vi "Write.vi"(8 "error in (no error)":errorcluster, 10 "Input":variant, 11 "DAQmx DIO in":refnum<class "DAQmx DIO.lvclass">) -> (0 "error out":errorcluster, 3 "DAQmx DIO out":refnum<class "DAQmx DIO.lvclass">)   [LabVIEW 2017, in "DAQmx DIO.lvclass"]
uses:
  DAQmx DIO.lvclass
  C:/Microcellular Plastics Lab/Hardware Settings/Hardware Types/DAQmx/DAQmx.lvclass
  DAQmx/DAQmx.lvclass/DAQmx.ctl
  <vilib>/DAQmx/write.llb/DAQmx Write (Digital 1D Bool NChan 1Samp 1Line).vi
  DAQmx/Accessors/Read DAQmx Task Name.vi
  <vilib>/DAQmx/miscellaneous.llb/DAQmx Fill In Error Info.vi
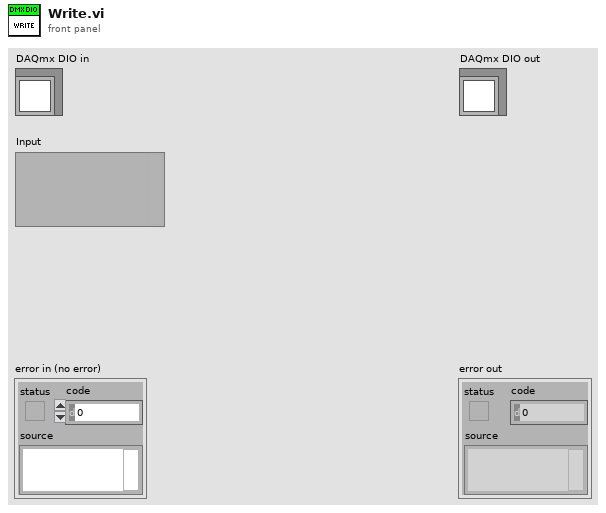
[diagram p1: front panel]
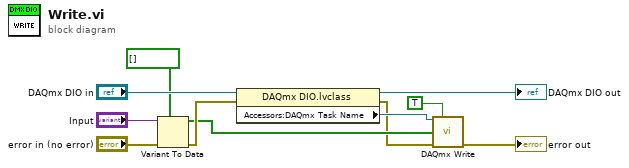
[diagram p0: block diagram]
diagram:
  n1 = Variant To Data(error in="error in (no error)", type=bool[] [], Variant="Input") -> (data=w3:bool[], error out=w7:errorcluster)
  n2 = property class="DAQmx DIO.lvclass"(reference="DAQmx DIO in", error in=w7) -> (reference out=→"DAQmx DIO out":refnum<class "DAQmx DIO.lvclass">, error out=w2:errorcluster, "Accessors:DAQmx Task Name"=w6:refnum<k21>)
  n3 = call-poly <vilib>:"DAQmx Write.vi"("task/channels in"=w6, "auto start"=TRUE, "data"=w3, "error in"=w2) -> ("error out"=→"error out":errorcluster)  [unwired: 9 in, 2 out]
